vi "Array of bluinking controllers.vi"(0 "Controls":refnum<vi>[](array[refnum]), 7 "Blinking":bool[](array[boolean]), 11 "error in":errorcluster) -> (15 "error out":errorcluster)   [LabVIEW 2011]
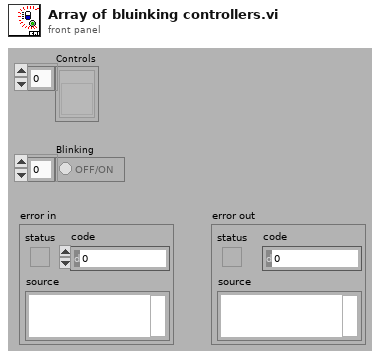
[diagram p1: front panel]
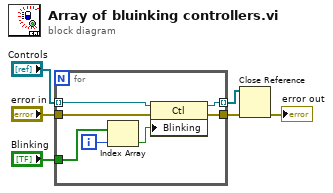
[diagram p0: block diagram]
diagram:
  n1 = for {
    tunnel: "error in" -> [w13]
    tunnel: [w12] -> w1
    tunnel: "Controls" -> [w11] mode=indexing
    tunnel: [w10] -> w2 mode=indexing
    tunnel: "Blinking" -> [w9]
    i -> [w8]
    n2 = Index Array(array=w9, index=w8) -> (element=w7:bool)
    n3 = property class="Ctl"(reference=w11, error in=w13, "Blinking"=w7) -> (reference out=w10:refnum<vi>, error out=w12:errorcluster)
  }
  n4 = Close Reference(reference=w2, error in (no error)=w1) -> (error out=→"error out":errorcluster)
